vi "Configure Modulation (Frequency-Shift Keying).vi"(6 "Shift Rate (10 Hz)":dbl=10.0, 7 "Enable Frequency-Shift Keying (T:Enable)":bool=TRUE, 8 "error in (no error)":errorcluster, 9 "FSK Alternate Frequency (100 Hz)":dbl=100.0, 10 "FSK Source (Internal)":enum16{"Internal", "External"}(ring), 11 "VISA resource name":refnum<visa-resource-name>) -> (0 "error out":errorcluster, 3 "VISA resource name out":refnum<visa-resource-name>)   [LabVIEW 2017, in "Keithley 3390.lvlib"]
doc: "Configures and enables frequency shift keying (FSK) modulation. In FSK, the frequency of the waveform is shifted between the carrier frequency and an alternate (\"Hop\") frequency. The shifting rate is determined by the modulating signal. \n\n<B>Note:</B> The carrier waveform shape and parameters are set by the Configure Waveform VI."
uses:
  Keithley 3390.lvlib
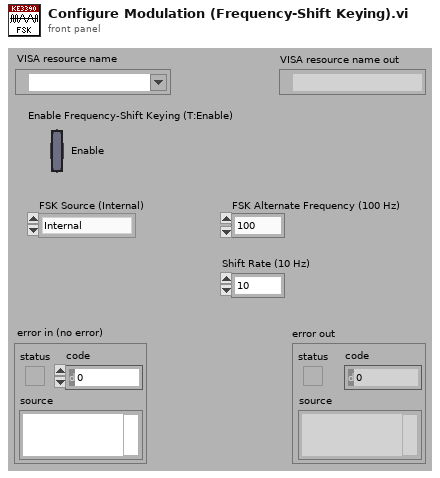
[diagram p1: front panel]
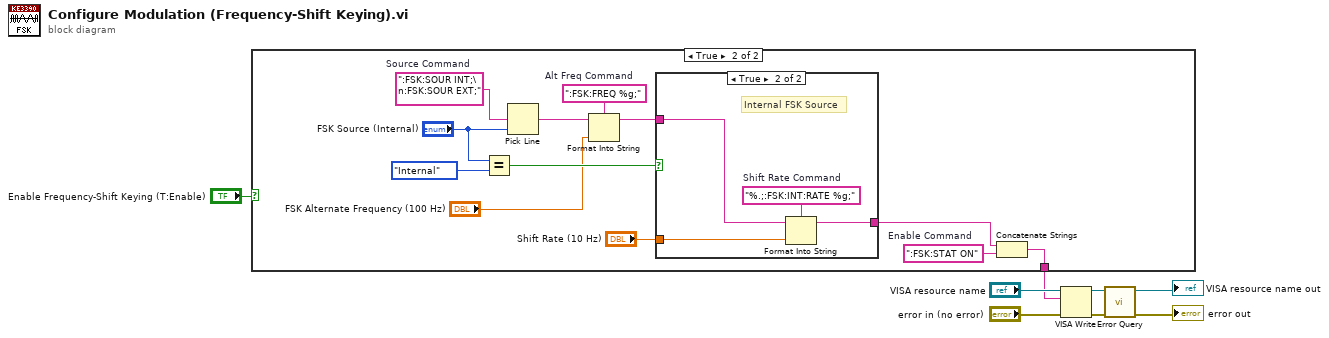
[diagram p0: block diagram]
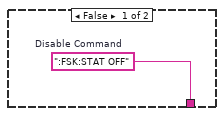
[diagram p2: hidden frame]
diagram:
  n1 = case shown="True" "Enable Frequency-Shift Keying (T:Enable)" {
    tunnel: [w9 w17] -> w6
    frame False {
      w9 = ":FSK:STAT OFF"  # Disable Command
    }
    frame True {
      w14 = ":FSK:FREQ %g;"  # Alt Freq Command
      w16 = ":FSK:STAT ON"  # Enable Command
      w20 = ":FSK:SOUR INT;\n:FSK:SOUR EXT;"  # Source Command
      n2 = Equal?(x="FSK Source (Internal)", y=enum16{"Internal", "External"}."Internal") -> (x = y?=w18:bool)
      n3 = Pick Line(multi-line string=w20, line index="FSK Source (Internal)") -> (output string=w12:string)  [unwired: 1 in]
      n4 = Format Into String(format string=w14, initial string=w12, "FSK Alternate Frequency (100 Hz)") -> (resulting string=w11:string)  [unwired: 1 in, 1 out]
      n5 = case shown="True" w18 {
        tunnel: [w22 w25] -> w10
        tunnel: "Shift Rate (10 Hz)" -> [_ w24]
        tunnel: w11 -> [w22 w23]
        frame False {
          # "External FSK Source"
        }
        frame True {
          w26 = "%.;:FSK:INT:RATE %g;"  # Shift Rate Command
          # "Internal FSK Source"
          n6 = Format Into String(format string=w26, initial string=w23, w24) -> (resulting string=w25:string)  [unwired: 1 in, 1 out]
        }
      }
      n7 = Concatenate Strings(w10, w16) -> (w17:string)
    }
  }
  n8 = VISA Write(VISA resource name="VISA resource name", write buffer=w6, error in (no error)="error in (no error)") -> (VISA resource name out=w4:refnum<visa-resource-name>, error out=w5:errorcluster)  [unwired: 1 out]
  n9 = call "Error Query.vi"("error in (no error)"=w5, "VISA resource name"=w4) -> ("error out"=→"error out":errorcluster, "VISA resource name out"=→"VISA resource name out":refnum<visa-resource-name>)  [unwired: 6 in, 2 out]
